vi "Write.Initialize.vi"(8 "error in":errorcluster, 10 "Custom Device API in":refnum<class "Custom Device API.lvclass">, 11 "Settings":cluster{"Refs":T1[], "Values":dbl[]} {"Refs"."Data Reference" format="%.0x"}) -> (0 "error out":errorcluster, 3 "Write out":refnum<class "Write.lvclass">)   [LabVIEW 2027, in "Data Access Engine (Express).lvlib" / "Write.lvclass"]
uses:
  Write.lvclass
  <vilib>/NI VeriStand/Custom Device API/Block Data Reference.ctl
  <vilib>/NI VeriStand/Custom Device API/Data Reference.ctl
  <userlib>/Custom Device Interfaces_v1.lvlibp/CustomDeviceAPI/Custom Device API.lvclass
  Write.lvclass/Write.ctl
  <vilib>/NI VeriStand/Custom Device API/Custom Device API.lvlib
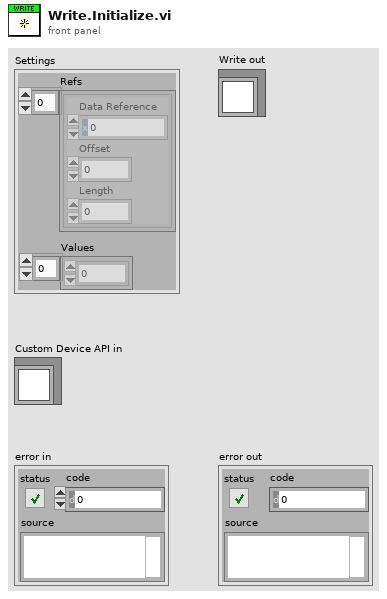
[diagram p1: front panel]
types:
  T1 = typedef "Custom Device API.lvlib/Block Data Reference.ctl" = cluster{"Data Reference":T2, "Offset":u64, "Length":u64}
  T2 = typedef "Custom Device API.lvlib/Data Reference.ctl" = i32
  T3 = cluster{"read mode":enum16{"polling", "blocking"}, "write mode":enum16{"polling", "blocking"}}
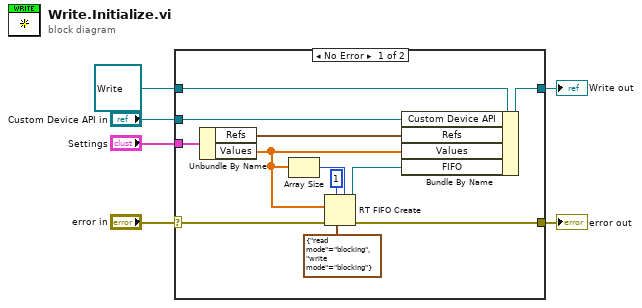
[diagram p0: block diagram]
diagram:
  n1 = case shown="No Error" "error in" {
    selector: "error in" -> [w11 w19]
    tunnel: [w18 w19] -> w6
    tunnel: refnum<class "Write.lvclass"> refnum ("Write in") -> [w13 w20]
    tunnel: [w12 w20] -> w4
    tunnel: "Settings" -> [w10 _]
    tunnel: "Custom Device API in" -> [w8 _]
    frame No Error {
      n2 = Unbundle By Name(w10) -> ("Refs"=w9:T1[], "Values"=w7:dbl[])
      n3 = Array Size(array=w7) -> (size(s)=w15:i32)
      n4 = RT FIFO Create(1:w7, 3:w11, 4:u32 1 ("size (10)"), 6:w15, 7:T3 {"read mode"=enum."blocking", "write mode"=enum."blocking"} ("r/w modes (polling,polling)")) -> (8:w17:refnum<k33>, 11:w18:errorcluster)  [unwired: 3 in, 1 out]
      n5 = Bundle By Name(cluster=w13, "Custom Device API"=w8, "Refs"=w9, "Values"=w7, "FIFO"=w17) -> (w12:refnum<class "Write.lvclass">)
    }
    frame Error {
    }
  }
  "error out" <- w6
  "Write out" <- w4
